vi "init.vi"(8 "error in (no error)":errorcluster, 10 "Pressure Sensor Settings":T1={"Channel"="", "Terminal Configuration"=10083, "Minimum"=-10.0, "Maximum"=10.0} {"Maximum" format="%.3f"; "Minimum" format="%.3f"; "Terminal Configuration" items=["Default"=-1, "RSE"=10083, "NRSE"=10078, "Differential"=10106, "Pseudodifferential"=12529]}, 11 "PressureSensor in":refnum<class "PressureSensor.lvclass">) -> (0 "error out":errorcluster, 3 "PressureSensor out":refnum<class "PressureSensor.lvclass">)   [LabVIEW 2015, in "PressureSensor.lvclass"]
uses:
  PressureSensor.lvclass
  Typedefs/Pressure Sensor Settings.ctl
  PressureSensor.lvclass/PressureSensor.ctl
  <vilib>/DAQmx/create/channels.llb/DAQmx Create Channel (AI-Voltage-Basic).vi
  Typedefs/FAMTTypedefs.lvlib
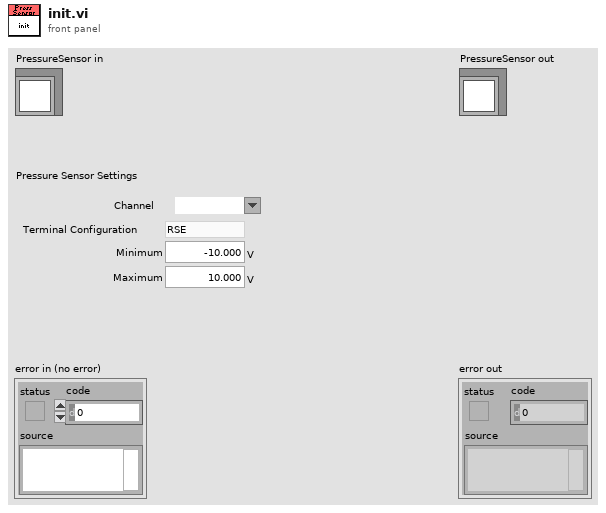
[diagram p1: front panel]
types:
  T1 = typedef "FAMTTypedefs.lvlib/Pressure Sensor Settings.ctl" = cluster{"Channel":tag, "Terminal Configuration":i32, "Minimum":dbl[unit], "Maximum":dbl[unit]}
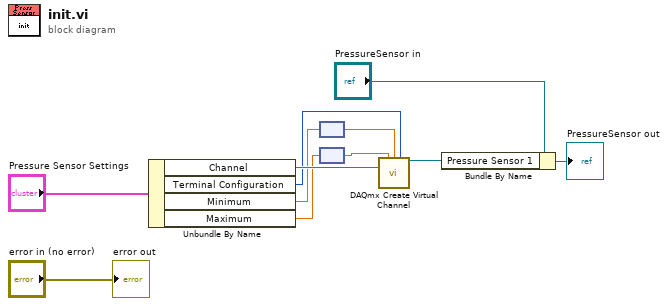
[diagram p0: block diagram]
diagram:
  n1 = Unbundle By Name("Pressure Sensor Settings") -> ("Channel"=w7:tag, "Terminal Configuration"=w6:i32, "Minimum"=w5:dbl[unit], "Maximum"=w3:dbl[unit])
  n2 = node(w5) -> (w4:dbl)
  n3 = node(w3) -> (w2:dbl)
  n4 = call-poly <vilib>:"DAQmx Create Virtual Channel.vi"("maximum value"=w2, "minimum value"=w4, "input terminal configuration"=w6, "physical channels"=w7) -> ("task out"=w1:refnum<k21>)  [unwired: 10 in, 1 out]
  n5 = Bundle By Name(cluster="PressureSensor in", "Pressure Sensor 1"=w1) -> (→"PressureSensor out":refnum<class "PressureSensor.lvclass">)
  "error out" <- "error in (no error)"
